vi "End Map.vi"   [LabVIEW 2018, in "Toolkit.lvlib" / "Reader.lvclass"]
doc: "Ends reading a map from the MessagePack data. This must be called after reading and decoding all key-value pairs in a map to avoid errors."
uses:
  Reader.lvclass
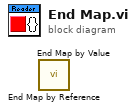
[diagram p0: block diagram]
diagram:
  n1 = call "End Map by Reference.vi"() -> ()  [unwired: 10 in, 2 out]
  n2 = call "End Map by Value.vi"() -> ()  [unwired: 10 in, 2 out]
